vi "frequency-table.vi"() -> (2 "value":i32[](array[numeric]))   [LabVIEW 2013]
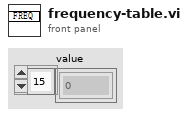
[diagram p1: front panel]
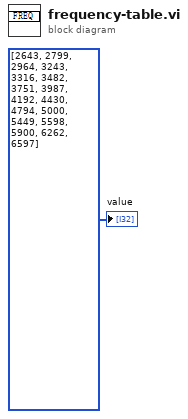
[diagram p0: block diagram]
diagram:
  "value" <- i32[] [2643, 2799, 2964, 3243, 3316, 3482, 3751, 3987, 4192, 4430, 4794, 5000, 5449, 5598, 5900, 6262, 6597] ("value")
